vi "Get Test cases Path.vi"() -> (1 "folder names":string[](array[string]), 2 "Array":path[](array[path]))   [LabVIEW 2021, in "Sequence Engine.lvlib" / "Test Factory.lvclass"]
uses:
  Test Factory.lvclass
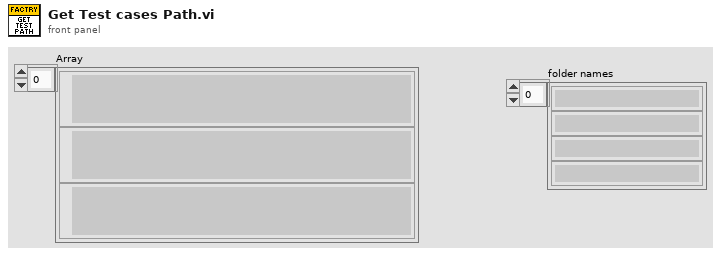
[diagram p1: front panel]
types:
  T1 = enum32{"invalid app kind", "Development System", "Run Time System", "Student Edition", "Embedded LabVIEW", "Evaluation", "Custom"}
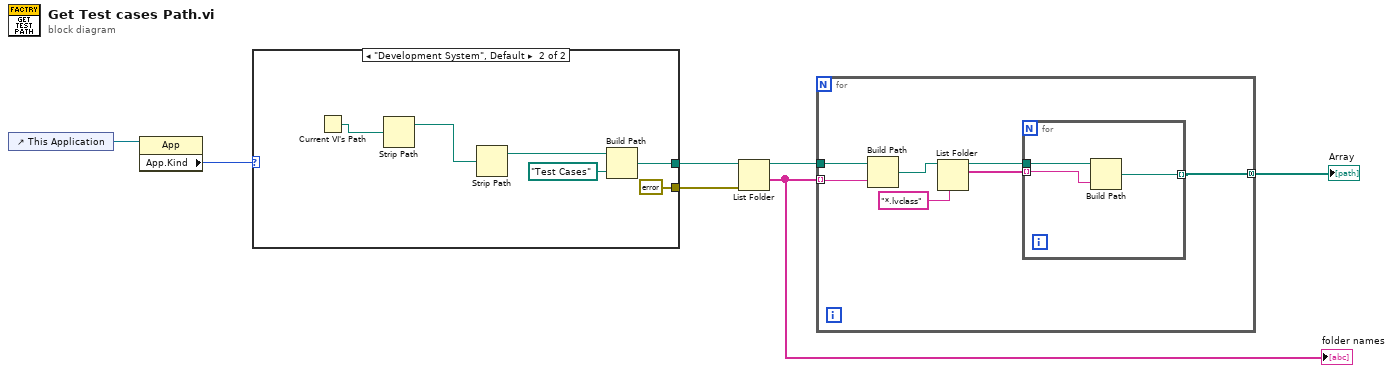
[diagram p0: block diagram]
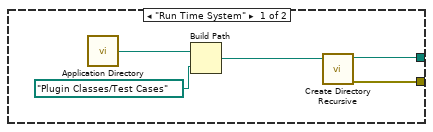
[diagram p2: hidden frame]
diagram:
  n1 = control-ref of="This Application"() -> (w2:refnum<vi>)
  n2 = property class="App"(reference=w2) -> ("App.Kind"=w1:T1)  [unwired: 1 in, 2 out]
  n3 = case shown="\"Development System\", Default" w1 {
    tunnel: [w9 w18] -> w4
    tunnel: [w8 errorcluster {"status"=FALSE, "code"=0, "source"=""} ("error out")] -> w3
    frame "Run Time System" {
      n4 = call <vilib>:"Application Directory.vi"() -> ("Application Directory"=w11:path)
      n5 = Build Path(base path=w11, name or relative path=path "Plugin Classes/Test Cases") -> (appended path=w10:path)
      n6 = call <vilib>:"Create Directory Recursive.vi"("directory"=w10) -> ("error out"=w8:errorcluster, "directory copy"=w9:path)  [unwired: 4 in, 1 out]
    }
    frame "Development System", Default {
      n7 = Current VI's Path() -> (path=w14:path)
      n8 = Strip Path(path=w14) -> (stripped path=w15:path)  [unwired: 1 out]
      n9 = Strip Path(path=w15) -> (stripped path=w16:path)  [unwired: 1 out]
      n10 = Build Path(base path=w16, name or relative path=path "Test Cases") -> (appended path=w18:path)
    }
  }
  n11 = List Folder(path=w4, error in=w3) -> (path out=w6:path, folder names=w5:string[])  [unwired: 2 in, 2 out]
  "folder names" <- w5
  n12 = for {
    tunnel: w5 -> [w24] mode=indexing
    tunnel: w6 -> [w25]
    tunnel: [w19] -> w7 mode=concatenating
    n13 = Build Path(base path=w25, name or relative path=w24) -> (appended path=w23:path)
    n14 = List Folder(path=w23, pattern="*.lvclass") -> (path out=w21:path, filenames=w20:string[])  [unwired: 2 in, 2 out]
    n15 = for {
      tunnel: w21 -> [w28]
      tunnel: w20 -> [w27] mode=indexing
      tunnel: [w26] -> w19 mode=indexing
      n16 = Build Path(base path=w28, name or relative path=w27) -> (appended path=w26:path)
    }
  }
  "Array" <- w7
